vi "Teleop.vi"(10 "Match Info":T1={"Autonomous Elapsed Seconds"=0.0, "TeleOp Elapsed Seconds"=126.441, "Disabled Elapsed Seconds"=32.205, "Visited Autonomous"=FALSE, "Visited TeleOp"=TRUE, "Visited Disabled"=TRUE, "Autonomous Settings"={"Autonomous Style"=enum."Independent", "VI Refnum"=refnum}}, 11 "Call Context":T2=enum."Execute") -> ()   [LabVIEW 2017]
doc: "This VI is called for each enabled TeleOp packet received from the DS. It is typically used to read from joysticks and other inputs and update I/O or setpoints for timed control loops. It should complete and return within 20 milliseconds or risk missing DS packets."
uses:
  <vilib>/Rock Robotics/WPI/DriverStation/WPI_DriverStationDerivedRobotMode.ctl
  <vilib>/Rock Robotics/WPI/DriverStation/WPI_DriverStationMatch Info.ctl
  <vilib>/Rock Robotics/WPI/Utilities/WPI_GetSetVariantRefNum.vi
  <vilib>/Rock Robotics/Network Tables/NT Write Boolean Array.vi
  <vilib>/Rock Robotics/Network Tables/NT Write Numeric Array.vi
  <vilib>/Rock Robotics/Network Tables/NT Write Number.vi
  Framework/Robot Global Data.vi
panel:
  in  "Turn Rate":dbl=0.75
  in  "Speed Rate":dbl=0.75
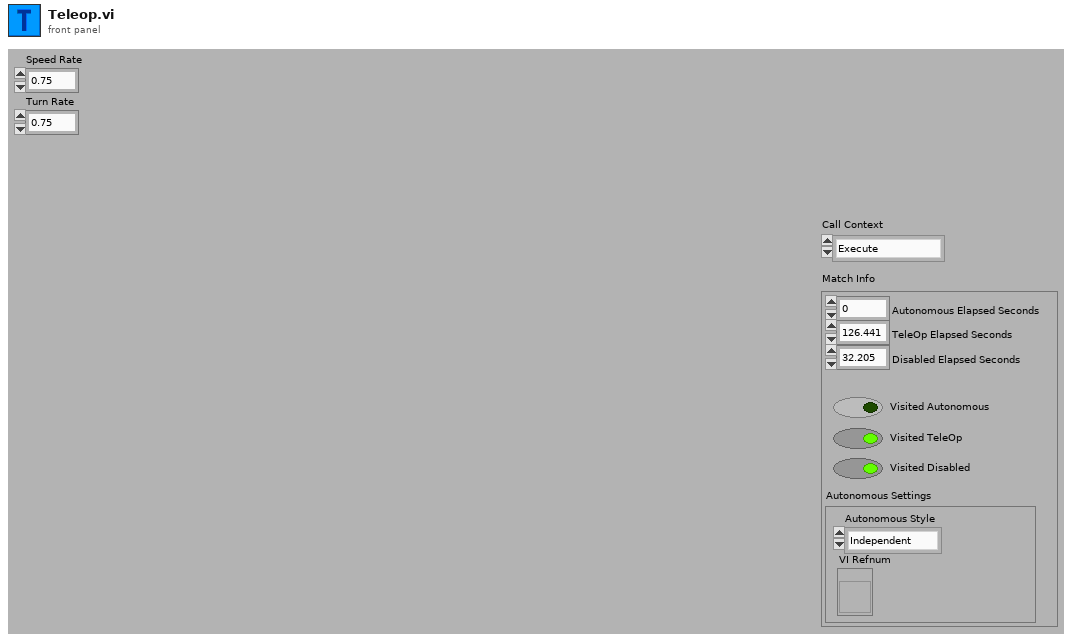
[diagram p1: front panel]
types:
  T1 = typedef "WPI_DriverStationMatch Info.ctl" = cluster{"Autonomous Elapsed Seconds":dbl, "TeleOp Elapsed Seconds":dbl, "Disabled Elapsed Seconds":dbl, "Visited Autonomous":bool, "Visited TeleOp":bool, "Visited Disabled":bool, "Autonomous Settings":cluster{"Autonomous Style":enum16{"Iterative", "Independent"}, "VI Refnum":refnum<vi>}}
  T2 = typedef "WPI_DriverStationDerivedRobotMode.ctl" = enum16{"Init", "Execute", "Stop"}
  T3 = cluster{"Grab Setpoint ":dbl, "Grab Time ":dbl, "Release Setpoint ":dbl, "Release Time ":dbl, " Button Lift Arm Setpoint ":dbl, "Button Lift Arm Time ":dbl, "Button Lower Arm Setpoint ":dbl, "Button Lower Arm Time ":dbl, "Climb Setpoint ":dbl, "Climb Time ":dbl, "Speed Rate ":dbl, "Speed Deadband ":dbl, "Turning Rate ":dbl, "Turning Deadband ":dbl}
  T4 = typedef "WPI_JoystickDevRef.ctl" = cluster{"Device":T5}
  T5 = typedef "WPI_JoystickDeviceEnum.ctl" = enum16{"USB 0", "USB 1", "USB 2", "USB 3", "USB 4", "USB 5"}
  T6 = typedef "Command Status Info.ctl" = cluster{"Name":string, "Status":T7, "notifier out":T8}
  T7 = typedef "Completion Status.ctl" = enum16{"Successful", "Aborted", "Incomplete"}
  T8 = typedef "Completion Notifier.ctl" = refnum<notifier>
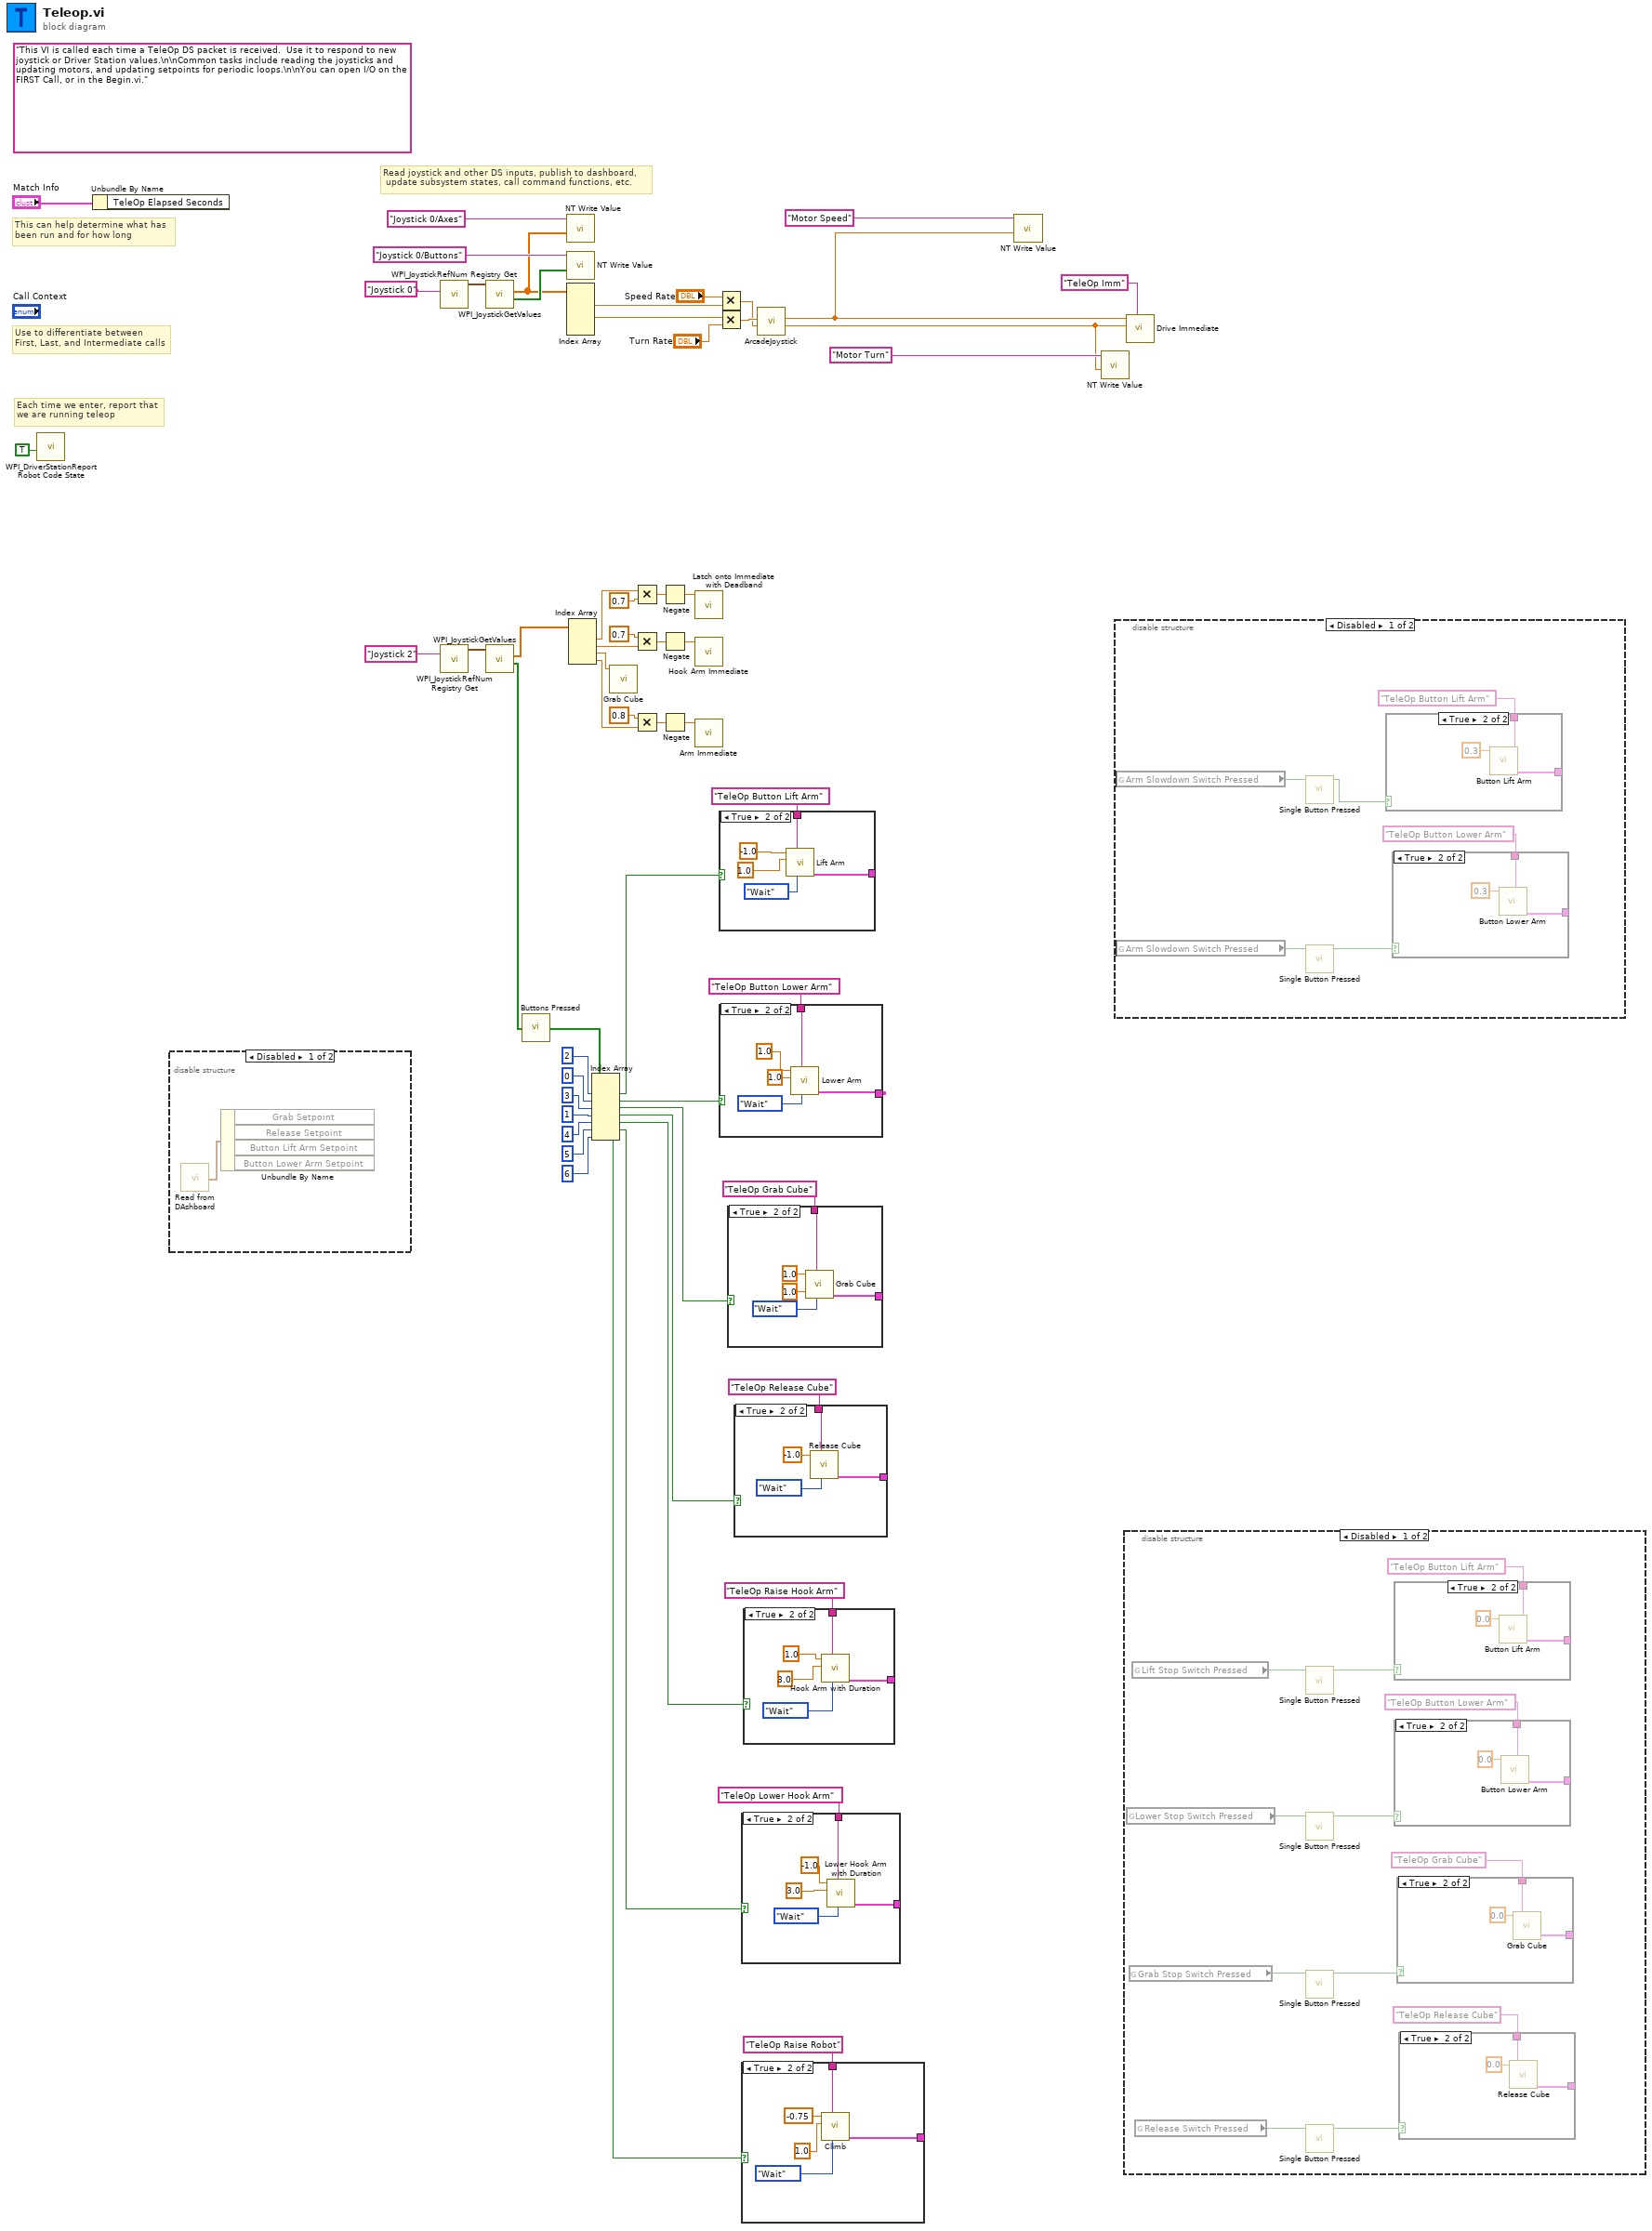
[diagram p0: block diagram]
diagram:
  (unwired) "This VI is called each time a TeleOp DS packet is received.  Use it to respond to new joystick or Driver Station values.\n\nCommon tasks include reading the joysticks and updating motors, and updating setpoints for periodic loops.\n\nYou can open I/O on the FIRST Call, or in the Begin.vi."
  # "Read joystick and other DS inputs, publish to dashboard,\n update subsystem states, call command functions, etc."
  # "Each time we enter, report that\nwe are running teleop"
  # "Use to differentiate between\nFirst, Last, and Intermediate calls"
  # "This can help determine what has\nbeen run and for how long"
  n1 = call <vilib>:"WPI_DriverStationReport Robot Code State.vi"("TeleOp"=TRUE ("Autonomous")) -> ()  [unwired: 10 in, 1 out]
  n2 = Unbundle By Name("Match Info") -> ()  [unwired: 1 out]
  n3 = disable-structure shown="Disabled" {
    frame Disabled {
      n4 = call "Read from DAshboard.vi"() -> ("output cluster"=w59:T3)  [unwired: 11 in]
      n5 = Unbundle By Name(w59) -> ()  [unwired: 4 out]
    }
    frame Enabled {
    }
  }
  n6 = call <vilib>:"WPI_JoystickRefNum Registry Get.vi"("refnum name"="Joystick 0") -> ("JoystickDevRef"=w55:T4)  [unwired: 1 in, 9 out]
  n7 = call <vilib>:"WPI_JoystickRefNum Registry Get.vi"("refnum name"="Joystick 2") -> ("JoystickDevRef"=w48:T4)  [unwired: 1 in, 9 out]
  n8 = call <vilib>:"WPI_JoystickGetValues.vi"("JoystickDevRef"=w55) -> ("Buttons"=w52:bool[], "Axes"=w51:dbl[])  [unwired: 6 in, 3 out]
  n9 = call <vilib>:"WPI_JoystickGetValues.vi"("JoystickDevRef"=w48) -> ("Buttons"=w15:bool[], "Axes"=w47:dbl[])  [unwired: 6 in, 3 out]
  n10 = call "Buttons Pressed.vi"("Button Values"=w15) -> ("Button Presses"=w39:bool[])
  n11 = call-poly <vilib>:"NT Write Value.vi"("Numeric Array"=w51, "Name"="Joystick 0/Axes") -> ()  [unwired: 9 in, 1 out]
  n12 = call-poly <vilib>:"NT Write Value.vi"("Boolean Array"=w52, "Name"="Joystick 0/Buttons") -> ()  [unwired: 9 in, 1 out]
  n13 = Index Array(array=w51) -> (element #2=w31:dbl, element #3=w30:dbl)  [unwired: 5 in, 3 out]
  n14 = Index Array(array=w47) -> (element #1=w3:dbl, element #2=w2:dbl, element #3=w34:dbl, element #4=w10:dbl)  [unwired: 4 in]
  n15 = Index Array(array=w39, index #1=2 ("index"), index #2=0 ("index"), index #3=3 ("index"), index #4=1 ("index"), index #5=4 ("index"), index #6=5 ("index"), index #7=6 ("index")) -> (element #1=w38:bool, element #2=w36:bool, element #3=w35:bool, element #4=w1:bool, element #5=w22:bool, element #6=w13:bool, element #7=w20:bool)
  n16 = call "Grab Cube.vi"("Setpoint"=w34) -> ()  [unwired: 10 in, 1 out]
  n17 = Multiply(x=w3, y=0.7 ("x")) -> (x*y=w7:dbl)
  n18 = Multiply(x=0.7, y=w2) -> (x*y=w8:dbl)
  n19 = Multiply(x=0.8, y=w10) -> (x*y=w46:dbl)
  n20 = Negate(x=w7) -> (-x=w5:dbl)
  n21 = Negate(x=w8) -> (-x=w6:dbl)
  n22 = Negate(x=w46) -> (-x=w44:dbl)
  n23 = call "Latch onto Immediate with Deadband.vi"("Setpoint"=w5) -> ()  [unwired: 10 in, 1 out]
  n24 = call "Hook Arm Immediate.vi"("Setpoint"=w6) -> ()  [unwired: 10 in, 1 out]
  n25 = call "Arm Immediate.vi"("Setpoint"=w44) -> ()  [unwired: 10 in, 1 out]
  n26 = Multiply(x="Speed Rate", y=w31) -> (x*y=w28:dbl)
  n27 = Multiply(x=w30, y="Turn Rate") -> (x*y=w29:dbl)
  n28 = case shown="True" w38 {
    tunnel: "TeleOp Button Lift Arm" ("Description") -> [_ w61]
    tunnel: [_ w62] -> _
    frame False {
    }
    frame True {
      n29 = call "Lift Arm.vi"("Synchronization"=enum16{"Start", "Wait"}."Wait", "Description"=w61, "Duration (s)"=1.0, "Setpoint"=-1.0) -> ("Command Info Out"=w62:T6)  [unwired: 7 in]
    }
  }
  n30 = case shown="True" w36 {
    tunnel: "TeleOp Button Lower Arm" ("Description") -> [_ w69]
    tunnel: [_ w66] -> _
    frame False {
    }
    frame True {
      n31 = call "Lower Arm.vi"("Synchronization"=enum16{"Start", "Wait"}."Wait", "Description"=w69, "Duration (s)"=1.0, "Setpoint"=1.0) -> ("Command Info Out"=w66:T6)  [unwired: 7 in]
    }
  }
  n32 = case shown="True" w35 {
    tunnel: "TeleOp Grab Cube" ("Description") -> [_ w74]
    tunnel: [_ w71] -> _
    frame False {
    }
    frame True {
      n33 = call "Grab Cube.vi"("Synchronization"=enum16{"Start", "Wait"}."Wait", "Description"=w74, "Duration (s)"=1.0, "Setpoint"=1.0) -> ("Command Info Out"=w71:T6)  [unwired: 7 in]
    }
  }
  n34 = case shown="True" w1 {
    tunnel: "TeleOp Release Cube" ("Description") -> [_ w78]
    tunnel: [_ w76] -> _
    frame False {
    }
    frame True {
      n35 = call "Release Cube.vi"("Synchronization"=enum16{"Start", "Wait"}."Wait", "Description"=w78, "Setpoint"=-1.0) -> ("Command Info Out"=w76:T6)  [unwired: 8 in]
    }
  }
  n36 = case shown="True" w13 {
    tunnel: "TeleOp Lower Hook Arm" ("Description") -> [_ w83]
    tunnel: [_ w80] -> _
    frame False {
    }
    frame True {
      n37 = call "Lower Hook Arm with Duration.vi"("Synchronization"=enum16{"Start", "Wait"}."Wait", "Description"=w83, "Duration (s)"=3.0, "Setpoint"=-1.0) -> ("Command Info Out"=w80:T6)  [unwired: 7 in]
    }
  }
  n38 = case shown="True" w20 {
    tunnel: "TeleOp Raise Robot" ("Description") -> [_ w88]
    tunnel: [_ w85] -> _
    frame False {
    }
    frame True {
      n39 = call "Climb.vi"("Synchronization"=enum16{"Start", "Wait"}."Wait", "Description"=w88, "Duration (s)"=1.0 ("x"), "Setpoint"=-0.75) -> ("Command Info Out"=w85:T6)  [unwired: 7 in]
    }
  }
  n40 = case shown="True" w22 {
    tunnel: "TeleOp Raise Hook Arm" ("Description") -> [_ w93]
    tunnel: [_ w90] -> _
    frame False {
    }
    frame True {
      n41 = call "Hook Arm with Duration.vi"("Synchronization"=enum16{"Start", "Wait"}."Wait", "Description"=w93, "Duration (s)"=3.0, "Setpoint"=1.0) -> ("Command Info Out"=w90:T6)  [unwired: 7 in]
    }
  }
  n42 = call "ArcadeJoystick.vi"("Y axis value"=w28, "X axis value"=w29) -> ("Right Motor Value"=w40:dbl, "Left Motor Value"=w41:dbl)  [unwired: 8 in]
  n43 = call-poly <vilib>:"NT Write Value.vi"("Numeric"=w41, "Name"="Motor Speed") -> ()  [unwired: 9 in, 1 out]
  n44 = call-poly <vilib>:"NT Write Value.vi"("Numeric"=w40, "Name"="Motor Turn") -> ()  [unwired: 9 in, 1 out]
  n45 = disable-structure shown="Disabled" {
    frame Disabled {
      n46 = global read "Robot Global Data.vi" "Arm Slowdown Switch Pressed"() -> (w99:bool)
      n47 = global read "Robot Global Data.vi" "Arm Slowdown Switch Pressed"() -> (w95:bool)
      n48 = call "Single Button Pressed.vi"("Button Value"=w99) -> ("Button Press"=w97:bool)  [unwired: 10 in]
      n49 = call "Single Button Pressed.vi"("Button Value"=w95) -> ("Button Press"=w94:bool)  [unwired: 10 in]
      n50 = case shown="True" w97 {
        tunnel: "TeleOp Button Lift Arm" ("Description") -> [_ w105]
        tunnel: [_ w104] -> _
        frame False {
        }
        frame True {
          n51 = call "Button Lift Arm.vi"("Description"=w105, "Setpoint"=0.3) -> ("Command Info Out"=w104:T6)  [unwired: 9 in]
        }
      }
      n52 = case shown="True" w94 {
        tunnel: "TeleOp Button Lower Arm" ("Description") -> [_ w102]
        tunnel: [_ w101] -> _
        frame False {
        }
        frame True {
          n53 = call "Button Lower Arm.vi"("Description"=w102, "Setpoint"=0.3) -> ("Command Info Out"=w101:T6)  [unwired: 9 in]
        }
      }
    }
    frame Enabled {
    }
  }
  n54 = disable-structure shown="Disabled" {
    frame Disabled {
      n55 = global read "Robot Global Data.vi" "Lower Stop Switch Pressed"() -> (w112:bool)
      n56 = global read "Robot Global Data.vi" "Grab Stop Switch Pressed"() -> (w111:bool)
      n57 = global read "Robot Global Data.vi" "Lift Stop Switch Pressed"() -> (w113:bool)
      n58 = global read "Robot Global Data.vi" "Release Switch Pressed"() -> (w110:bool)
      n59 = call "Single Button Pressed.vi"("Button Value"=w113) -> ("Button Press"=w106:bool)  [unwired: 10 in]
      n60 = call "Single Button Pressed.vi"("Button Value"=w112) -> ("Button Press"=w107:bool)  [unwired: 10 in]
      n61 = call "Single Button Pressed.vi"("Button Value"=w111) -> ("Button Press"=w108:bool)  [unwired: 10 in]
      n62 = call "Single Button Pressed.vi"("Button Value"=w110) -> ("Button Press"=w109:bool)  [unwired: 10 in]
      n63 = case shown="True" w106 {
        tunnel: "TeleOp Button Lift Arm" ("Description") -> [_ w129]
        tunnel: [_ w128] -> _
        frame False {
        }
        frame True {
          n64 = call "Button Lift Arm.vi"("Description"=w129, "Setpoint"=0.0) -> ("Command Info Out"=w128:T6)  [unwired: 9 in]
        }
      }
      n65 = case shown="True" w107 {
        tunnel: "TeleOp Button Lower Arm" ("Description") -> [_ w126]
        tunnel: [_ w125] -> _
        frame False {
        }
        frame True {
          n66 = call "Button Lower Arm.vi"("Description"=w126, "Setpoint"=0.0) -> ("Command Info Out"=w125:T6)  [unwired: 9 in]
        }
      }
      n67 = case shown="True" w108 {
        tunnel: "TeleOp Grab Cube" ("Description") -> [_ w123]
        tunnel: [_ w122] -> _
        frame False {
        }
        frame True {
          n68 = call "Grab Cube.vi"("Description"=w123, "Setpoint"=0.0) -> ("Command Info Out"=w122:T6)  [unwired: 9 in]
        }
      }
      n69 = case shown="True" w109 {
        tunnel: "TeleOp Release Cube" ("Description") -> [_ w120]
        tunnel: [_ w119] -> _
        frame False {
        }
        frame True {
          n70 = call "Release Cube.vi"("Description"=w120, "Setpoint"=0.0) -> ("Command Info Out"=w119:T6)  [unwired: 9 in]
        }
      }
    }
    frame Enabled {
    }
  }
  n71 = call "Drive Immediate.vi"("Description"="TeleOp Imm", "Right Setpoint"=w40, "Left Setpoint"=w41) -> ()  [unwired: 8 in, 1 out]
